vi "saveDocument.vi"(8 "error in (no error)":errorcluster, 10 "Document Path":path, 11 "npoiDocument in":refnum<class "npoiDocument.lvclass">) -> (0 "error out":errorcluster, 3 "npoiDocument out":refnum<class "npoiDocument.lvclass">)   [LabVIEW 2017, in "NPOI_Document.lvlib" / "npoiDocument.lvclass"]
uses:
  npoiDocument.lvclass
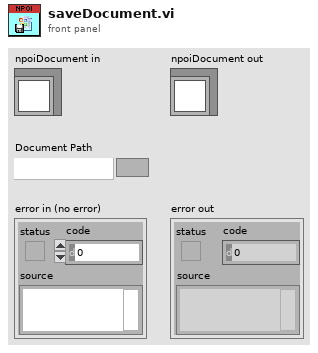
[diagram p1: front panel]
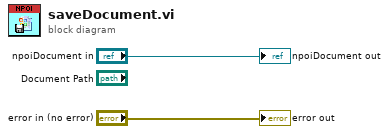
[diagram p0: block diagram]
diagram:
  "error out" <- "error in (no error)"
  "npoiDocument out" <- "npoiDocument in"
